vi "Test Digital Output.vi"(8 "error in":errorcluster, 10 "TestCase in":refnum<class "Scan Engine Scripting API Modules.lvclass">, 11 "module test in":refnum<class "Module Test.lvclass">) -> (0 "error out":errorcluster, 2 "TestCase out":refnum<class "Scan Engine Scripting API Modules.lvclass">, 3 "module test out":refnum<class "Module Test.lvclass">)   [LabVIEW 2017, in "Module Test.lvclass"]
uses:
  Module Test.lvclass
  Scan Engine Scripting API Modules.lvclass
  C:/Program Files (x86)/National Instruments/LabVIEW 2017/vi.lib/addons/_JKI Toolkits/VI Tester/TestCase.llb/TestCase.lvclass
  Scripting/Modules/Mode Classes/Controls/digital channel settings.ctl
  Module Test.lvclass/Module Test.ctl
  Scripting/Scan Engine Scripting.lvlib
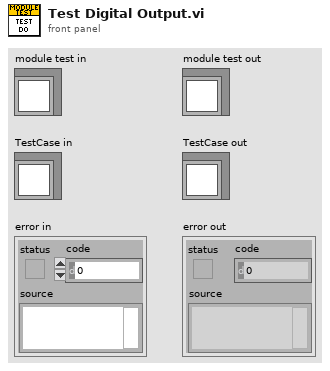
[diagram p1: front panel]
types:
  T1 = typedef "Scan Engine Scripting.lvlib/digital channel settings.ctl" = cluster{"name":string, "default value":bool}
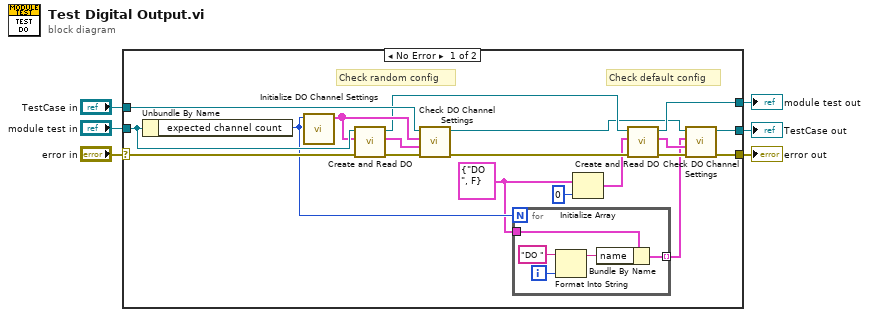
[diagram p0: block diagram]
diagram:
  n1 = case shown="No Error" "error in" {
    selector: "error in" -> [w22 w33]
    tunnel: [w16 w33] -> w5
    tunnel: [w17 w32] -> w3
    tunnel: "module test in" -> [w25 w32]
    tunnel: "TestCase in" -> [w24 w31]
    tunnel: [w13 w31] -> w1
    frame No Error {
      w8 = T1 {"name"="DO ", "default value"=FALSE} ("channel settings")
      # "Check default config"
      # "Check random config"
      n2 = Unbundle By Name(w25) -> ("expected channel count"=w10:i32)
      n3 = call "Initialize DO Channel Settings.vi"("array size"=w10) -> ("channel settings"=w23:T1[])  [unwired: 10 in]
      n4 = call-dynamic "Create and Read DO.vi"("error in"=w22, "initial channel settings"=w23, "module test in"=w25) -> ("error out"=w21:errorcluster, "read channel settings"=w20:T1[], "module test out"=w19:refnum<class "Module Test.lvclass">)  [unwired: 6 in]
      n5 = call "Check DO Channel Settings.vi"("error in"=w21, "read channel settings"=w20, "initial channel settings"=w23, "TestCase in"=w24) -> ("error out"=w18:errorcluster, "TestCase out"=w14:refnum<class "Scan Engine Scripting API Modules.lvclass">)  [unwired: 6 in]
      n6 = for {
        N: w10 -> [_]
        tunnel: [w27] -> w11 mode=indexing
        tunnel: w8 -> [w26]
        i -> [w30]
        n7 = Format Into String(initial string="DO ", w30) -> (resulting string=w28:string)  [unwired: 2 in, 1 out]
        n8 = Bundle By Name(cluster=w26, "name"=w28) -> (w27:T1)
      }
      n9 = Initialize Array(w8, 0 ("dimension size")) -> (w7:T1[])
      n10 = call-dynamic "Create and Read DO.vi"("error in"=w18, "initial channel settings"=w7, "module test in"=w19) -> ("error out"=w15:errorcluster, "read channel settings"=w12:T1[], "module test out"=w17:refnum<class "Module Test.lvclass">)  [unwired: 6 in]
      n11 = call "Check DO Channel Settings.vi"("error in"=w15, "read channel settings"=w12, "initial channel settings"=w11, "TestCase in"=w14) -> ("error out"=w16:errorcluster, "TestCase out"=w13:refnum<class "Scan Engine Scripting API Modules.lvclass">)  [unwired: 6 in]
    }
    frame Error {
    }
  }
  "error out" <- w5
  "module test out" <- w3
  "TestCase out" <- w1
